vi "Ideal Gas.vi"(7 "Data":T1) -> (0 "Simulation Objects":refnum<class "SimulationObject.lvclass">[](array[class]), 1 "Cell Size":i16, 2 "Gravity Vector out":refnum<class "Vector2.lvclass">, 3 "Background Color out":u32(colorbox))   [LabVIEW 2022 SP3]
uses:
  Engine/Math/Vector2/Vector2.lvclass
  Engine/Objects/SimulationObject/SimulationObject.lvclass
  Engine/Math/Vector2/Vector2.lvclass/Vector2.ctl
  Engine/Objects/SimulationObject/SimulationObject.lvclass/SimulationObject.ctl
  Engine/Objects/Components/PhysicsComponent/PhysicsComponent.lvclass/PhysicsComponent.ctl
  <vilib>/numeric/Random Number (Range) I64.vi
  Engine/Math/Vector2/Read x.vi
  Engine/Math/Vector2/Read y.vi
  <vilib>/numeric/sub_Random U32.vi
  Engine/Objects/Shapes/CircleShape/CircleShape.lvclass
  D:/Programowanie/Studia/Labview/CollisionSimulator/Project/Engine/Objects/Shapes/Shapeable/Shapeable.lvclass
  Engine/Objects/Shapes/RectangleShape/RectangleShape.lvclass
  Engine/Objects/Components/PhysicsComponent/PhysicsComponent.lvclass
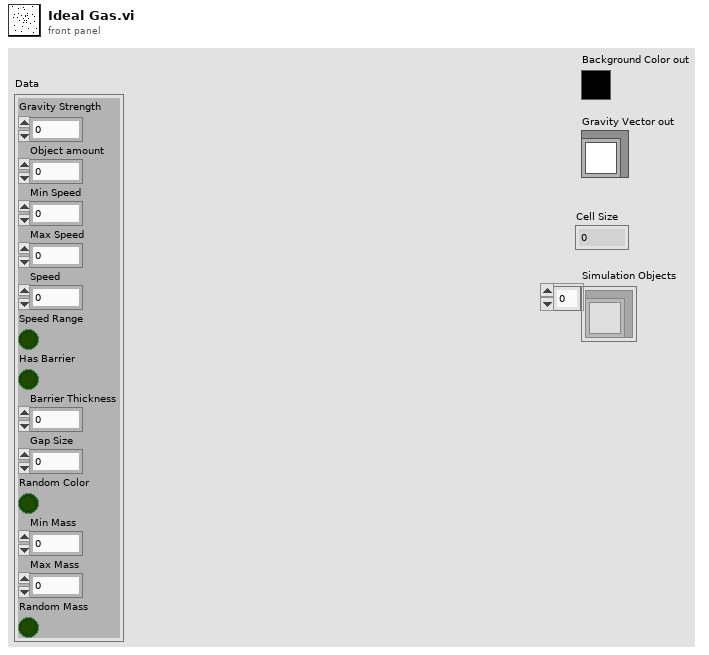
[diagram p1: front panel]
types:
  T1 = cluster{"Gravity Strength":sgl, "Object amount":dbl, "Min Speed":dbl, "Max Speed":dbl, "Speed":dbl, "Speed Range":bool, "Has Barrier":bool, "Barrier Thickness":dbl, "Gap Size":dbl, "Random Color":bool, "Min Mass":dbl, "Max Mass":dbl, "Random Mass":bool}
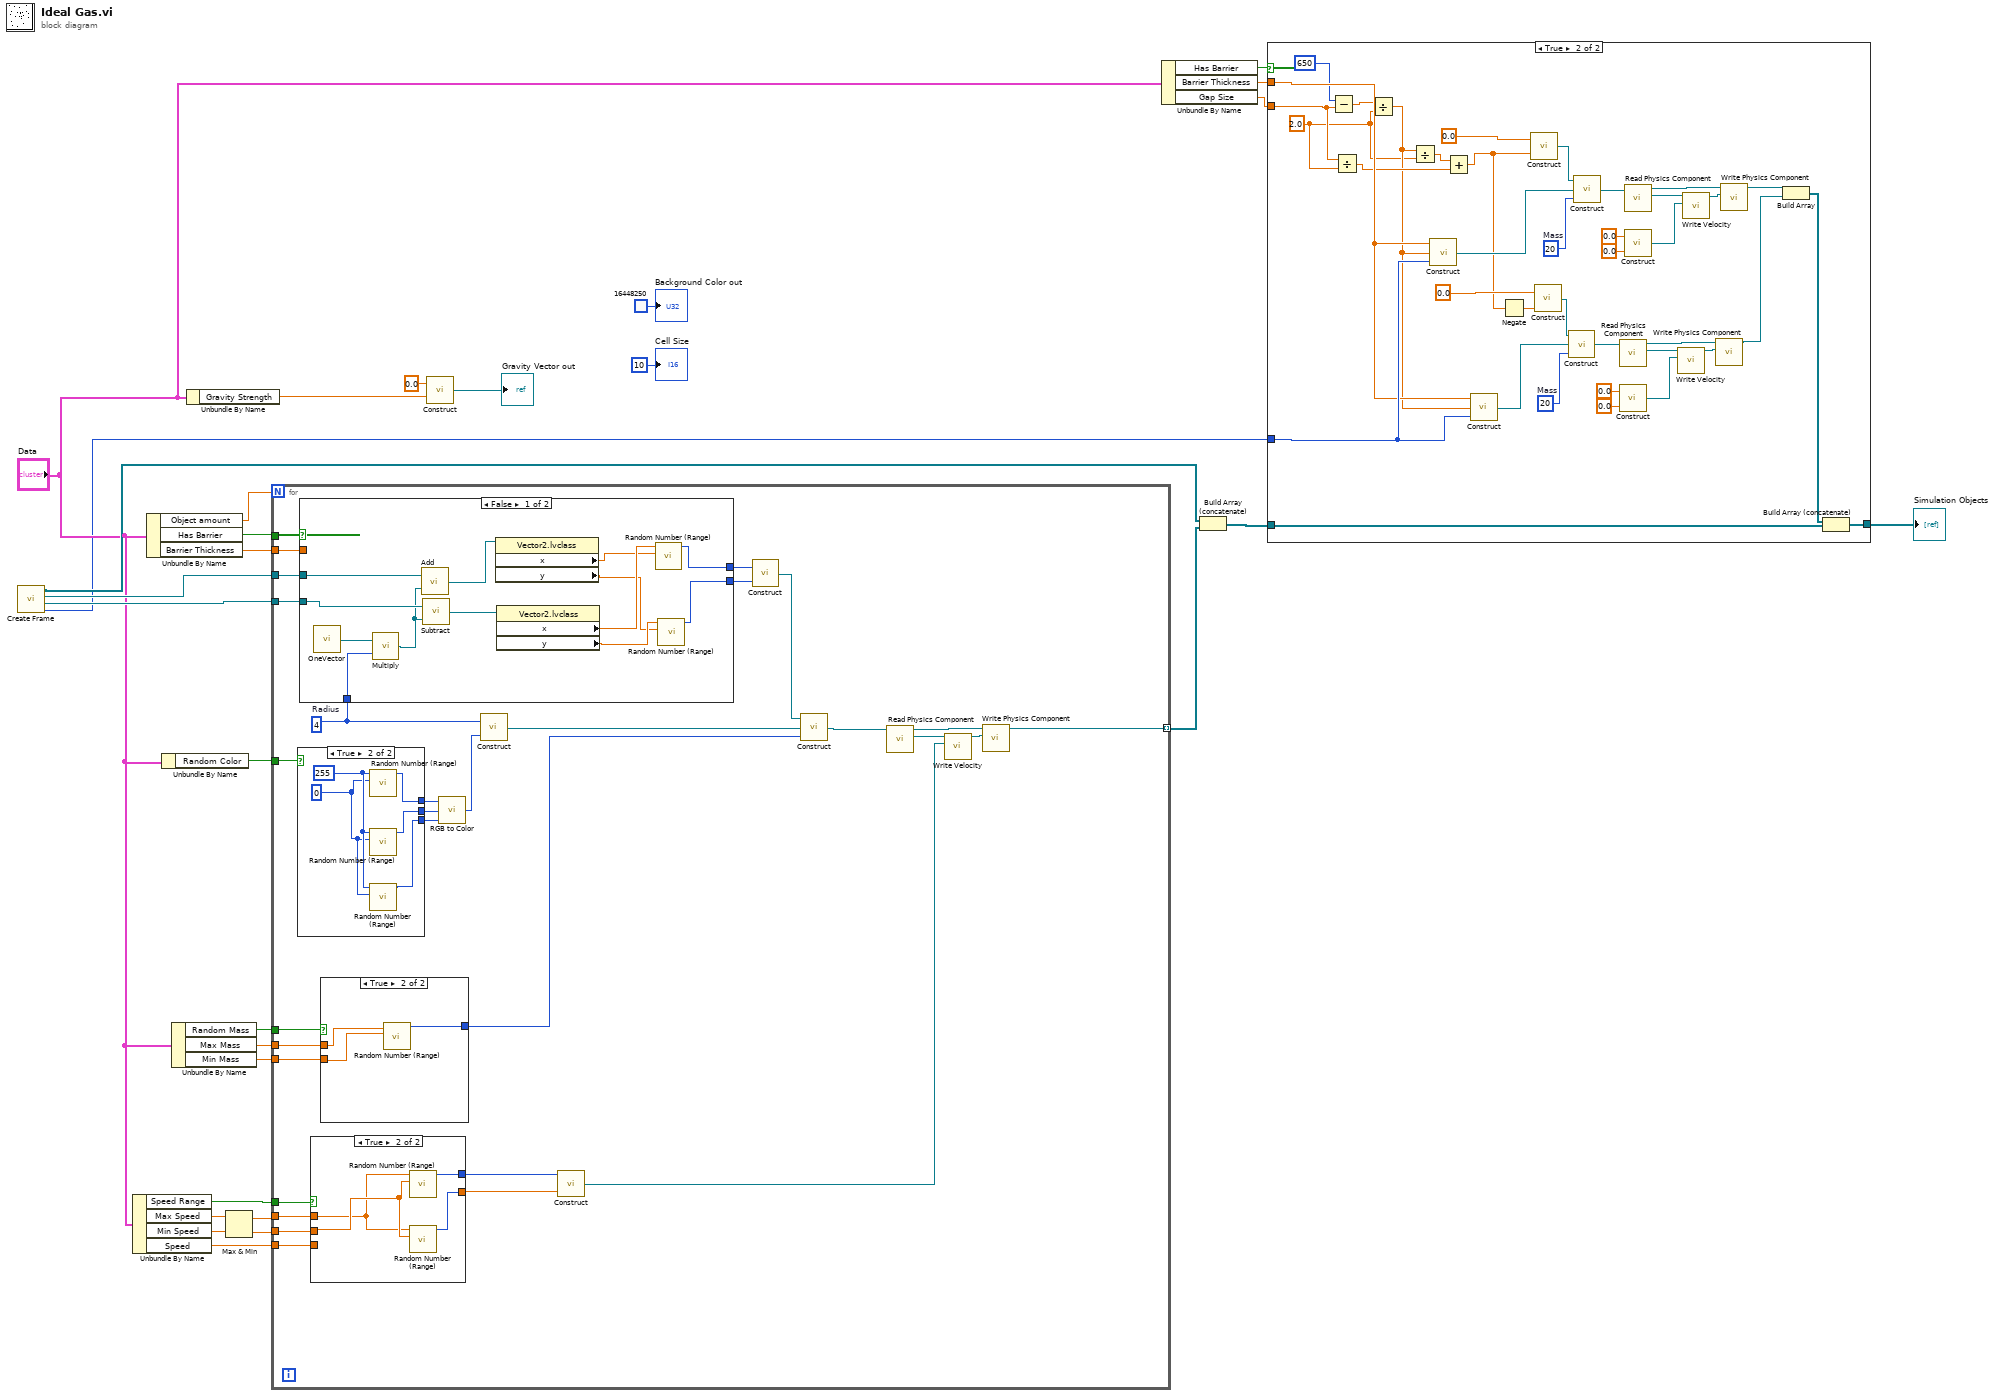
[diagram p0: block diagram]
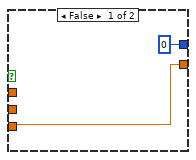
[diagram p3: hidden frame]
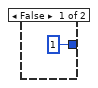
[diagram p4: hidden frame]
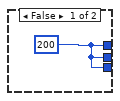
[diagram p5: hidden frame]
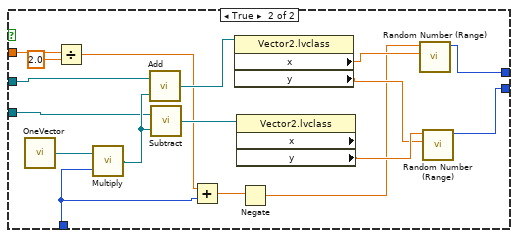
[diagram p6: hidden frame]
diagram:
  n1 = call "Create Frame.vi"() -> ("Color"=w3:u32, "Max Available Position"=w21:refnum<class "Vector2.lvclass">, "Min Available Position"=w22:refnum<class "Vector2.lvclass">, "Simulation Objects"=w10:refnum<class "SimulationObject.lvclass">[])  [unwired: 4 in]
  n2 = Unbundle By Name("Data") -> ("Speed Range"=w16:bool, "Max Speed"=w14:dbl, "Min Speed"=w13:dbl, "Speed"=w15:dbl)
  n3 = Unbundle By Name("Data") -> ("Object amount"=w24:dbl, "Has Barrier"=w23:bool, "Barrier Thickness"=w7:dbl)
  n4 = Unbundle By Name("Data") -> ("Random Color"=w20:bool)
  n5 = Unbundle By Name("Data") -> ("Random Mass"=w19:bool, "Max Mass"=w18:dbl, "Min Mass"=w17:dbl)
  n6 = Unbundle By Name("Data") -> ("Gravity Strength"=w28:sgl)
  n7 = Max & Min(x=w14, y=w13) -> (max(x,y)=w12:dbl, min(x,y)=w11:dbl)
  n8 = for {
    N: w24 -> [_]
    tunnel: w23 -> [w51]
    tunnel: w22 -> [w30]
    tunnel: w21 -> [w50]
    tunnel: w20 -> [w46]
    tunnel: w19 -> [w42]
    tunnel: w18 -> [w41]
    tunnel: w17 -> [w40]
    tunnel: w16 -> [w36]
    tunnel: w11 -> [w35]
    tunnel: w12 -> [w34]
    tunnel: w15 -> [w33]
    tunnel: [w32] -> w9 mode=indexing
    tunnel: w7 -> [w31]
    w49 = 4  # Radius
    n9 = case shown="True" w46 {
      tunnel: [w70 w73] -> w45
      tunnel: [w70 w72] -> w44
      tunnel: [w70 w71] -> w43
      frame False {
        w70 = i64 200 ("number")
      }
      frame True {
        w74 = 0
        w75 = 255
        n10 = call-poly <vilib>:"Random Number (Range).vi"("lower bound (-100)"=w74, "upper bound (100)"=w75) -> ("number"=w73:i64)  [unwired: 9 in]
        n11 = call-poly <vilib>:"Random Number (Range).vi"("lower bound (-100)"=w74, "upper bound (100)"=w75) -> ("number"=w72:i64)  [unwired: 9 in]
        n12 = call-poly <vilib>:"Random Number (Range).vi"("lower bound (-100)"=w74, "upper bound (100)"=w75) -> ("number"=w71:i64)  [unwired: 9 in]
      }
    }
    n13 = case shown="False" w51 {
      tunnel: w50 -> [w85 w97]
      tunnel: w49 -> [w87 w91]
      tunnel: [w77 w95] -> w48
      tunnel: [w76 w96] -> w47
      tunnel: w31 -> [_ w94]
      tunnel: w30 -> [w86 w98]
      frame False {
        n14 = call "OneVector.vi"() -> ("One Vector"=w88:refnum<class "Vector2.lvclass">)
        n15 = call "Multiply.vi"("Scalar"=w87, "Vector in"=w88) -> ("Vector out"=w84:refnum<class "Vector2.lvclass">)
        n16 = call "Add.vi"("Vec2 b in"=w84, "Vec2 a in"=w86) -> ("Vec2 out"=w83:refnum<class "Vector2.lvclass">)
        n17 = call "Subtract.vi"("Vec2 b in"=w84, "Vec2 a in"=w85) -> ("Vec2 out"=w82:refnum<class "Vector2.lvclass">)
        n18 = property class="Vector2.lvclass"(reference=w83) -> ("x"=w80:sgl, "y"=w78:sgl)  [unwired: 1 in, 2 out]
        n19 = property class="Vector2.lvclass"(reference=w82) -> ("x"=w81:sgl, "y"=w79:sgl)  [unwired: 1 in, 2 out]
        n20 = call-poly <vilib>:"Random Number (Range).vi"("lower bound (-100)"=w80, "upper bound (100)"=w81) -> ("number"=w77:i64)  [unwired: 9 in]
        n21 = call-poly <vilib>:"Random Number (Range).vi"("lower bound (-100)"=w78, "upper bound (100)"=w79) -> ("number"=w76:i64)  [unwired: 9 in]
      }
      frame True {
        n22 = call "OneVector.vi"() -> ("One Vector"=w105:refnum<class "Vector2.lvclass">)
        n23 = Divide(x=w94, y=2.0) -> (x/y=w92:dbl)
        n24 = call "Multiply.vi"("Scalar"=w91, "Vector in"=w105) -> ("Vector out"=w104:refnum<class "Vector2.lvclass">)
        n25 = call "Add.vi"("Vec2 b in"=w104, "Vec2 a in"=w98) -> ("Vec2 out"=w103:refnum<class "Vector2.lvclass">)
        n26 = call "Subtract.vi"("Vec2 b in"=w104, "Vec2 a in"=w97) -> ("Vec2 out"=w102:refnum<class "Vector2.lvclass">)
        n27 = Add(x=w92, y=w91) -> (x+y=w90:dbl)
        n28 = property class="Vector2.lvclass"(reference=w103) -> ("x"=w101:sgl, "y"=w99:sgl)  [unwired: 1 in, 2 out]
        n29 = property class="Vector2.lvclass" props=["x", "y"](reference=w102) -> ("y"=w100:sgl)  [unwired: 1 in, 3 out]
        n30 = Negate(x=w90) -> (-x=w89:dbl)
        n31 = call-poly <vilib>:"Random Number (Range).vi"("lower bound (-100)"=w101, "upper bound (100)"=w89) -> ("number"=w95:i64)  [unwired: 9 in]
        n32 = call-poly <vilib>:"Random Number (Range).vi"("lower bound (-100)"=w99, "upper bound (100)"=w100) -> ("number"=w96:i64)  [unwired: 9 in]
      }
    }
    n33 = case shown="True" w36 {
      tunnel: [w61 w65] -> w37
      tunnel: [i64 0 ("number") w64] -> w38
      tunnel: w35 -> [_ w63]
      tunnel: w34 -> [_ w62]
      tunnel: w33 -> [w61 _]
      frame False {
      }
      frame True {
        n34 = call-poly <vilib>:"Random Number (Range).vi"("lower bound (-100)"=w63, "upper bound (100)"=w62) -> ("number"=w64:i64)  [unwired: 9 in]
        n35 = call-poly <vilib>:"Random Number (Range).vi"("lower bound (-100)"=w63, "upper bound (100)"=w62) -> ("number"=w65:i64)  [unwired: 9 in]
      }
    }
    n36 = case shown="True" w42 {
      tunnel: w41 -> [_ w69]
      tunnel: w40 -> [_ w68]
      tunnel: [i64 1 ("number") w67] -> w39
      frame False {
      }
      frame True {
        n37 = call-poly <vilib>:"Random Number (Range).vi"("lower bound (-100)"=w68, "upper bound (100)"=w69) -> ("number"=w67:i64)  [unwired: 9 in]
      }
    }
    n38 = call <vilib>:"RGB to Color.vi"("B"=w43, "G"=w44, "R"=w45) -> ("Color"=w53:u32)
    n39 = call "Construct.vi"("Color"=w53, "Radius"=w49) -> ("CircleShape out"=w52:refnum<class "CircleShape.lvclass">)
    n40 = call "Construct.vi"("y"=w37, "x"=w38) -> ("Vec2 out"=w54:refnum<class "Vector2.lvclass">)
    n41 = call "Construct.vi"("y"=w47, "x"=w48) -> ("Vec2 out"=w59:refnum<class "Vector2.lvclass">)
    n42 = call "Construct.vi"("Mass"=w39, "Shape in"=w52, "Local Position in"=w59) -> ("Simulation Object out"=w58:refnum<class "SimulationObject.lvclass">)
    n43 = call "Read Physics Component.vi"("SimulationObject in"=w58) -> ("Physics Component out"=w55:refnum<class "PhysicsComponent.lvclass">, "SimulationObject out"=w57:refnum<class "SimulationObject.lvclass">)  [unwired: 8 in, 1 out]
    n44 = call "Write Velocity.vi"("Velocity in"=w54, "PhysicsComponent in"=w55) -> ("PhysicsComponent out"=w56:refnum<class "PhysicsComponent.lvclass">)  [unwired: 8 in, 1 out]
    n45 = call "Write Physics Component.vi"("PhysicsComponent.lvclass"=w56, "SimulationObject in"=w57) -> ("SimulationObject out"=w32:refnum<class "SimulationObject.lvclass">)  [unwired: 8 in, 1 out]
  }
  n46 = call "Construct.vi"("y"=w28, "x"=sgl 0.0) -> ("Vec2 out"=→"Gravity Vector out":refnum<class "Vector2.lvclass">)
  n47 = Unbundle By Name("Data") -> ("Has Barrier"=w6:bool, "Barrier Thickness"=w2:dbl, "Gap Size"=w1:dbl)
  n48 = Build Array (concatenate)(w10, w9) -> (w5:refnum<class "SimulationObject.lvclass">[])
  n49 = case shown="True" w6 {
    tunnel: w5 -> [w106 w118]
    tunnel: [w106 w119] -> w4
    tunnel: w3 -> [_ w121]
    tunnel: w2 -> [_ w120]
    tunnel: w1 -> [_ w108]
    frame False {
    }
    frame True {
      w107 = 2.0 ("y")
      w124 = 20  # Mass
      w128 = 20  # Mass
      n50 = Subtract(x=650, y=w108) -> (x-y=w115:dbl)
      n51 = Divide(x=w108, y=w107) -> (x/y=w114:dbl)
      n52 = Divide(x=w115, y=w107) -> (x/y=w109:dbl)
      n53 = Divide(x=w109, y=w107) -> (x/y=w110:dbl)
      n54 = call "Construct.vi"("Color"=w121, "Height"=w109, "Width"=w120) -> ("RectangleShape out"=w135:refnum<class "RectangleShape.lvclass">)
      n55 = Add(x=w110, y=w114) -> (x+y=w111:dbl)
      n56 = call "Construct.vi"("Color"=w121, "Height"=w109, "Width"=w120) -> ("RectangleShape out"=w136:refnum<class "RectangleShape.lvclass">)
      n57 = Negate(x=w111) -> (-x=w113:dbl)
      n58 = call "Construct.vi"("y"=w111, "x"=sgl 0.0) -> ("Vec2 out"=w134:refnum<class "Vector2.lvclass">)
      n59 = call "Construct.vi"("y"=w113, "x"=sgl 0.0) -> ("Vec2 out"=w137:refnum<class "Vector2.lvclass">)
      n60 = call "Construct.vi"("Mass"=w124, "Shape in"=w136, "Local Position in"=w137) -> ("Simulation Object out"=w138:refnum<class "SimulationObject.lvclass">)
      n61 = call "Construct.vi"("Mass"=w128, "Shape in"=w135, "Local Position in"=w134) -> ("Simulation Object out"=w133:refnum<class "SimulationObject.lvclass">)
      n62 = call "Read Physics Component.vi"("SimulationObject in"=w138) -> ("Physics Component out"=w141:refnum<class "PhysicsComponent.lvclass">, "SimulationObject out"=w139:refnum<class "SimulationObject.lvclass">)  [unwired: 8 in, 1 out]
      n63 = call "Construct.vi"("y"=sgl 0.0, "x"=sgl 0.0) -> ("Vec2 out"=w142:refnum<class "Vector2.lvclass">)
      n64 = call "Read Physics Component.vi"("SimulationObject in"=w133) -> ("Physics Component out"=w130:refnum<class "PhysicsComponent.lvclass">, "SimulationObject out"=w132:refnum<class "SimulationObject.lvclass">)  [unwired: 8 in, 1 out]
      n65 = call "Construct.vi"("y"=sgl 0.0, "x"=sgl 0.0) -> ("Vec2 out"=w129:refnum<class "Vector2.lvclass">)
      n66 = call "Write Velocity.vi"("Velocity in"=w142, "PhysicsComponent in"=w141) -> ("PhysicsComponent out"=w140:refnum<class "PhysicsComponent.lvclass">)  [unwired: 8 in, 1 out]
      n67 = call "Write Velocity.vi"("Velocity in"=w129, "PhysicsComponent in"=w130) -> ("PhysicsComponent out"=w131:refnum<class "PhysicsComponent.lvclass">)  [unwired: 8 in, 1 out]
      n68 = call "Write Physics Component.vi"("PhysicsComponent.lvclass"=w140, "SimulationObject in"=w139) -> ("SimulationObject out"=w144:refnum<class "SimulationObject.lvclass">)  [unwired: 8 in, 1 out]
      n69 = call "Write Physics Component.vi"("PhysicsComponent.lvclass"=w131, "SimulationObject in"=w132) -> ("SimulationObject out"=w143:refnum<class "SimulationObject.lvclass">)  [unwired: 8 in, 1 out]
      n70 = Build Array(w143, w144) -> (w117:refnum<class "SimulationObject.lvclass">[])
      n71 = Build Array (concatenate)(w117, w118) -> (w119:refnum<class "SimulationObject.lvclass">[])
    }
  }
  "Simulation Objects" <- w4
  "Background Color out" <- u32 16448250 ("Background Color out")
  "Cell Size" <- i16 10 ("Cell Size")
